vi "Read Criteria.vi"(11 "UniquenessCriteria in":refnum<class "UniquenessCriteria.lvclass">) -> (2 "Criteria":T1, 3 "UniquenessCriteria out":refnum<class "UniquenessCriteria.lvclass">)   [LabVIEW 2014, in "UniquenessCriteria.lvclass"]
uses:
  UniquenessCriteria.lvclass
  Criteria.ctl
  UniquenessCriteria.lvclass/UniquenessCriteria.ctl
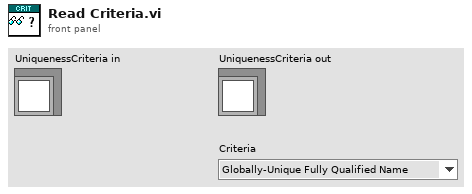
[diagram p1: front panel]
types:
  T1 = typedef "UniquenessCriteria.lvclass/Criteria.ctl" = enum16{"Globally-Unique Fully Qualified Name", "Globally-Unique Name"}
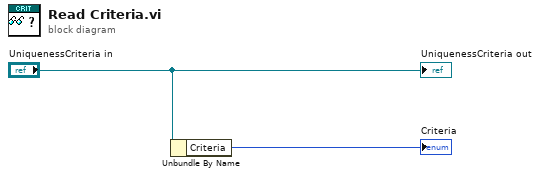
[diagram p0: block diagram]
diagram:
  n1 = Unbundle By Name("UniquenessCriteria in") -> ("Criteria"=→"Criteria":T1)
  "UniquenessCriteria out" <- "UniquenessCriteria in"
